vi "BRig_Host_dataRunState_dataTS_LorR.vi"() -> (2 "output_idx_dataTS_LorR":i32)   [LabVIEW 2014]
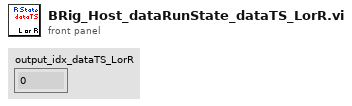
[diagram p1: front panel]
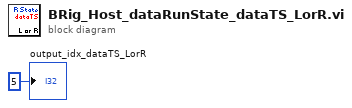
[diagram p0: block diagram]
diagram:
  "output_idx_dataTS_LorR" <- 5 ("output_idx_dataTS")
